vi "SendProgram.vi"(0 "Type of scan":u16, 1 "Line Axis":i32=1 min=1 max=4, 2 "Avg Num":i32=1, 4 "lines per scan plane":u16=128, 5 "Reverse ?":bool, 6 "Therapy/AVG ?":bool, 9 "File Names":string[](array[string]), 10 "I/O chan for motor pulse":i32=7, 19 "Offset":sgl) -> (15 "Error Status":bool)   [LabVIEW 2022 SP3]
uses:
  -MotionRoutines/MotionGlobals.vi
panel:
  in  "Min trig repeat time (s)":dbl=0.01
  out "MM2000 Response":string
  # "allows movement down axis where pulse is sent out every time Step to Move has\nbeen moved. Small program is sent to MM2000 and executed. Motion is kind of slow."
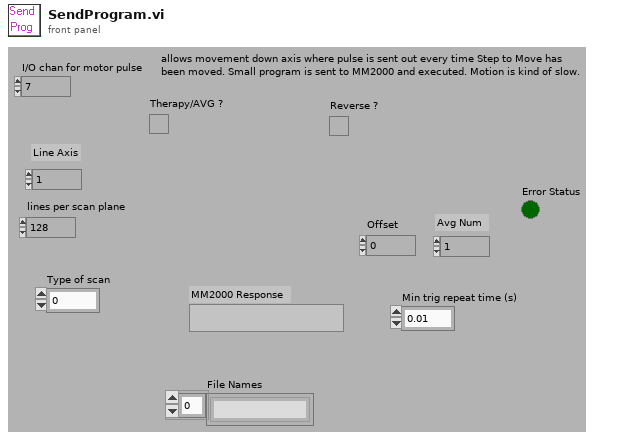
[diagram p1: front panel]
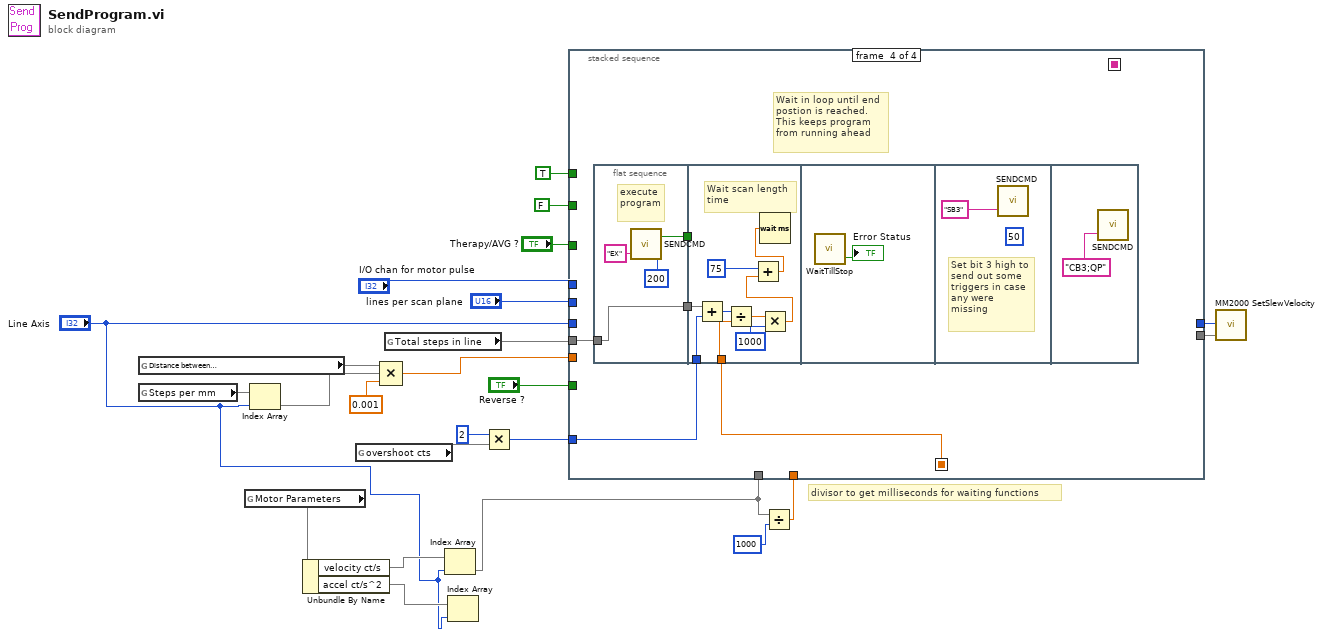
[diagram p0: block diagram]
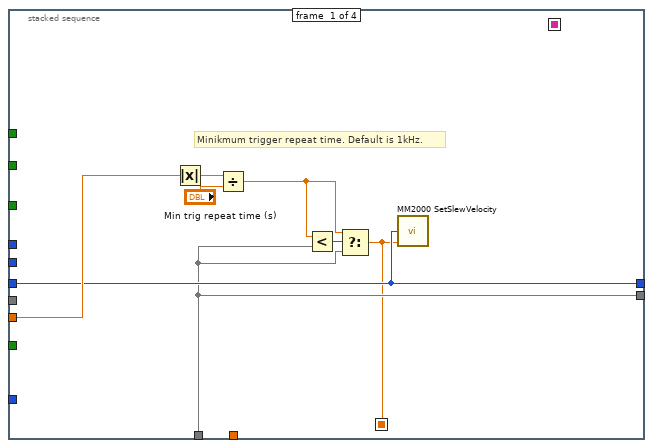
[diagram p2: hidden frame]
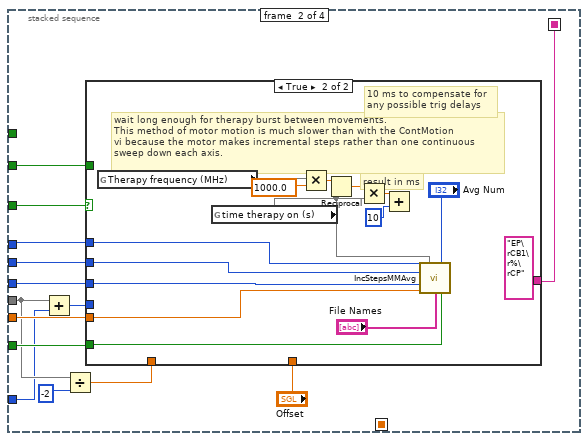
[diagram p3: hidden frame]
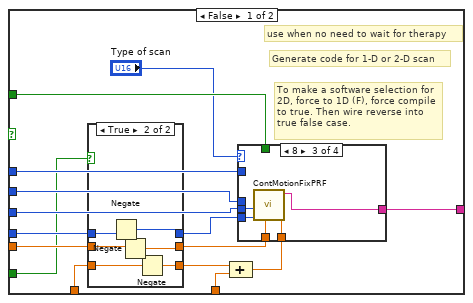
[diagram p4: hidden frame]
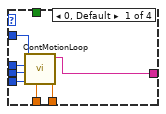
[diagram p5: hidden frame]
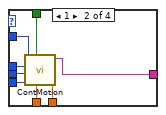
[diagram p6: hidden frame]
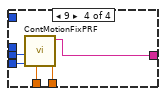
[diagram p7: hidden frame]
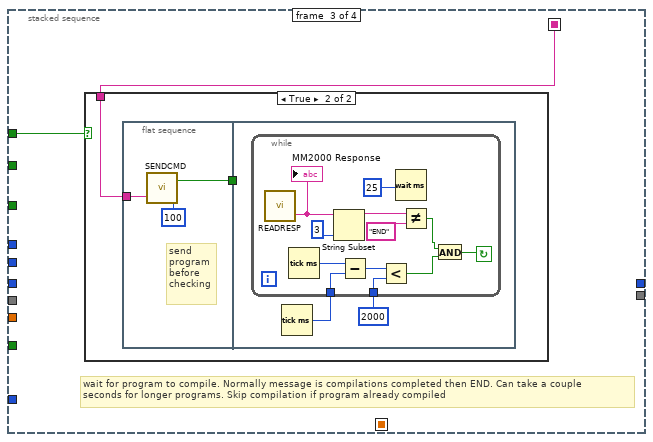
[diagram p9: hidden frame]
diagram:
  # "divisor to get milliseconds for waiting functions"
  n1 = global read "MotionGlobals.vi" "Distance between\nscan lines (mm)"() -> (w8)
  n2 = global read "MotionGlobals.vi" "Steps per mm"() -> (w10)
  n3 = global read "MotionGlobals.vi" "Motor Parameters"() -> (w3)
  n4 = Index Array(array=w10, index="Line Axis") -> (element=w6)
  n5 = Unbundle By Name(w3) -> ("velocity ct/s"=w5, "accel ct/s^2"=w4)
  n6 = global read "MotionGlobals.vi" "overshoot cts"() -> (w14)
  n7 = Compound Arithmetic op=MULTIPLY(w8, w6, 0.001) -> (w7:dbl)
  n8 = global read "MotionGlobals.vi" "Total steps in line"() -> (w11)
  n9 = Index Array(array=w5, index="Line Axis") -> (element=w1)
  n10 = Index Array(array=w4, index="Line Axis") -> ()  [unwired: 1 out]
  n11 = Multiply(x=2, y=w14) -> (x*y=w12:i32)
  n12 = Divide(x=w1, y=1000) -> (x/y=w19:dbl)
  n13 = stacked-sequence {
    seq-local: [_ w42 _ _] -> [_ _ w111 _]
    seq-local: [w25 _ _ _] -> [_ _ _ w132]
    tunnel: w11 -> [_ w35 _ w134]
    tunnel: "I/O chan for motor pulse" -> [_ w41 _ _]
    tunnel: w7 -> [w28 w43 _ _]
    tunnel: "Line Axis" -> [w27 w46 _ _]
    tunnel: "lines per scan plane" -> [_ w45 _ _]
    tunnel: "Therapy/AVG ?" -> [_ w44 _ _]
    tunnel: TRUE -> [_ _ w112 _]
    tunnel: "Reverse ?" -> [_ w40 _ _]
    tunnel: w19 -> [_ _ _ _]
    tunnel: w1 -> [w26 _ _ _]
    tunnel: [w27 _ _ _] -> w18
    tunnel: [w26 _ _ _] -> w17
    tunnel: FALSE -> [_ w39 _ _]
    tunnel: w12 -> [_ w33 _ w133]
    frame #0 {
      # "Minikmum trigger repeat time. Default is 1kHz."
      n14 = Absolute Value(x=w28) -> (abs(x)=w31:dbl)
      n15 = Divide(x=w31, y="Min trig repeat time (s)") -> (x/y=w30:dbl)
      n16 = Less?(x=w30, y=w26) -> (x < y?=w32:bool)
      n17 = Select(t=w30, s=w32, f=w26) -> (s? t:f=w25:dbl)
      n18 = call "MM2000 SetSlewVelocity.vi"("Slew Velocity"=w25, "Axis"=w27) -> ()  [unwired: 1 in]
    }
    frame #1 {
      n19 = Add(x=w35, y=w33) -> (x+y=w38:i32)
      n20 = Divide(x=w35, y=-2) -> (x/y=w34:dbl)
      n21 = case shown="True" w44 {
        tunnel: [w58 "EP\rCB1\r%\rCP"] -> w42
        tunnel: w41 -> [w59 w98]
        tunnel: w43 -> [w55 w110]
        tunnel: w46 -> [w61 w109]
        tunnel: w45 -> [w60 w108]
        tunnel: w38 -> [w57 _]
        tunnel: w40 -> [w52 w97]
        tunnel: w39 -> [w56 _]
        tunnel: "Offset" -> [w50 _]
        tunnel: w34 -> [w49 _]
        frame False {
          # "To make a software selection for 2D, force to 1D (F), force compile to true. Then wire reverse into true false case."
          # "use when no need to wait for therapy"
          # "Generate code for 1-D or 2-D scan"
          n22 = case shown="True" w52 {
            tunnel: [w89 w95] -> w53
            tunnel: w57 -> [w89 w92]
            tunnel: [w88 w94] -> w54
            tunnel: w55 -> [w88 w93]
            tunnel: [w87 w90] -> w48
            tunnel: w49 -> [w87 w91]
            frame False {
            }
            frame True {
              n23 = Negate(x=w92) -> (-x=w95:i32)
              n24 = Negate(x=w93) -> (-x=w94:dbl)
              n25 = Negate(x=w91) -> (-x=w90:dbl)
            }
          }
          n26 = Compound Arithmetic op=ADD(w48, w50) -> (w51:sgl)
          n27 = case shown="8" "Type of scan" {
            tunnel: w61 -> [w68 w76 w81 w86]
            tunnel: w60 -> [w67 w75 _ _]
            tunnel: w59 -> [w66 w74 _ _]
            tunnel: [w65 w73 w80 w85] -> w58
            tunnel: w56 -> [_ w72 _ _]
            tunnel: w51 -> [w64 w71 w79 w84]
            tunnel: w54 -> [w63 w70 w78 w83]
            tunnel: w53 -> [w62 w69 w77 w82]
            frame 0, Default {
              n28 = call "ContMotionLoop.vi"("Offset"=w64, "steps between scans"=w63, "total steps in line"=w62, "Axis"=w68, "lines per scan"=w67, "I/O chan for motor pulse"=w66) -> ("Output String"=w65:string)  [unwired: 1 in, 4 out]
            }
            frame 1 {
              n29 = call "ContMotion.vi"("Offset"=w71, "steps between scans"=w70, "1-D (F) 2-D (T)"=w72, "total steps in line"=w69, "Axis"=w76, "lines per scan"=w75, "I/O chan for motor pulse"=w74) -> ("Output String"=w73:string)  [unwired: 1 in, 3 out]
            }
            frame 8 {
              n30 = call "ContMotionFixPRF.vi"("Offset"=w79, "steps between scans"=w78, "total steps in line"=w77, "Axis"=w81) -> ("Output String"=w80:string)  [unwired: 3 in, 4 out]
            }
            frame 9 {
              n31 = call "ContMotionFixPRF.vi"("Offset"=w84, "steps between scans"=w83, "total steps in line"=w82, "Axis"=w86) -> ("Output String"=w85:string)  [unwired: 3 in, 4 out]
            }
          }
        }
        frame True {
          # "10 ms to compensate for\nany possible trig delays"
          # "wait long enough for therapy burst between movements.\nThis method of motor motion is much slower than with the ContMotion\nvi because the motor makes incremental steps rather than one continuous\nsweep down each axis."
          # "result in ms"
          n32 = global read "MotionGlobals.vi" "Therapy frequency (MHz)"() -> (w105)
          n33 = global read "MotionGlobals.vi" "time therapy on (s)"() -> (w99)
          n34 = Multiply(x=w105, y=1000.0) -> (x*y=w104:dbl)
          n35 = Reciprocal(x=w104) -> (1/x=w107:dbl)
          n36 = Multiply(x=w107, y=w99) -> (x*y=w103:dbl)
          n37 = Add(x=w103, y=10) -> ()  [unwired: 1 out]
          n38 = call "IncStepsMMAvg.vi"("I/O chan for motor pulse"=w98, "wait time between scans (ms)"=w99, "Avg Num"="Avg Num", "number of scans"=w108, "Axis"=w109, "Steps to move"=w110, "Crate File Names"="File Names", "Reverse ?"=w97) -> ()  [unwired: 2 in, 6 out]
        }
      }
    }
    frame #2 {
      # "wait for program to compile. Normally message is compilations completed then END. Can take a couple \nseconds for longer programs. Skip compilation if program already compiled"
      n39 = case shown="True" w112 {
        tunnel: w111 -> [_ w114]
        frame False {
        }
        frame True {
          n40 = flat-sequence {
            tunnel: w114 -> [w116]
            tunnel: [w115] -> w113
            tunnel: w113 -> [_]
            frame #0 {
              # "send\nprogram\nbefore\nchecking"
              n41 = call "SENDCMD.VI"("Wait time (ms)"=100, "MM2000 Command (ASCII String)"=w116) -> ("Boolean"=w115:bool)  [unwired: 1 in]
            }
            frame #1 {
              n42 = Tick Count (ms)() -> (millisecond timer value=w119:u32)
              n43 = while {
                tunnel: w119 -> [w126]
                tunnel: 2000 -> [w124]
                stop <- w121 continue-if-true
                n44 = call "READRESP.VI"() -> ("MM2000 Response (ASCII String)"=w120:string)  [unwired: 1 in]
                "MM2000 Response" <- w120
                n45 = Tick Count (ms)() -> (millisecond timer value=w127:u32)
                n46 = String Subset(string=w120, length (rest)=3) -> (substring=w130:string)  [unwired: 1 out]
                n47 = Subtract(x=w127, y=w126) -> (x-y=w125:u32)
                n48 = Less?(x=w125, y=w124) -> (x < y?=w122:bool)
                n49 = Wait (ms)(milliseconds to wait=25) -> ()  [unwired: 1 out]
                n50 = Not Equal?(x=w130, y="END") -> (x != y?=w123:bool)
                n51 = And(x=w123, y=w122) -> (x .and. y?=w121:bool)
              }
            }
          }
        }
      }
    }
    frame #3 {
      # "Wait in loop until end postion is reached. This keeps program from running ahead"
      n52 = flat-sequence {
        tunnel: [w138] -> w136
        tunnel: [w137] -> w135
        tunnel: w134 -> [w137]
        tunnel: w136 -> [_]
        tunnel: w135 -> [w148]
        tunnel: w132 -> [w144]
        tunnel: w133 -> [w149]
        frame #0 {
          # "execute program"
          n53 = call "SENDCMD.VI"("Wait time (ms)"=200, "MM2000 Command (ASCII String)"="EX") -> ("Boolean"=w138:bool)  [unwired: 1 in]
        }
        frame #1 {
          # "Wait scan length\ntime"
          n54 = Add(x=w148, y=w149) -> (x+y=w145:i32)
          n55 = Divide(x=w145, y=w144) -> (x/y=w147:dbl)
          n56 = Multiply(x=w147, y=1000) -> (x*y=w143:dbl)
          n57 = Add(x=75, y=w143) -> (x+y=w142:dbl)
          n58 = Wait (ms)(milliseconds to wait=w142) -> ()  [unwired: 1 out]
        }
        frame #2 {
          n59 = call "WaitTillStop.vi"() -> ("Error Status"=→"Error Status":bool)  [unwired: 3 out]
        }
        frame #3 {
          (unwired) 50
          # "Set bit 3 high to send out some triggers in case any were missing"
          n60 = call "SENDCMD.VI"("MM2000 Command (ASCII String)"="SB3") -> ()  [unwired: 2 in, 1 out]
        }
        frame #4 {
          n61 = call "SENDCMD.VI"("MM2000 Command (ASCII String)"="CB3;QP") -> ()  [unwired: 2 in, 1 out]
        }
      }
    }
  }
  n62 = call "MM2000 SetSlewVelocity.vi"("Slew Velocity"=w17, "Axis"=w18) -> ()  [unwired: 1 in]
